vi "demo_Plug-in Open Source Library.vi"(11 "Stop Demo":refnum<user-event>) -> ()   [LabVIEW 2020]
panel:
  # "Open Source Library for FlexLogger Plug-ins\n\nA variety of community and NI contributed useful plug-ins written in LabVIEW for extending your FlexLogger Pro experience\n\nUse what's there or contribute your own!\n\nLook for 'Sequencer with Output Values' in FlexLogger Sessions\n\nhttps://github.com/ni/niflexlogger-plugins/tree/main/plugins"
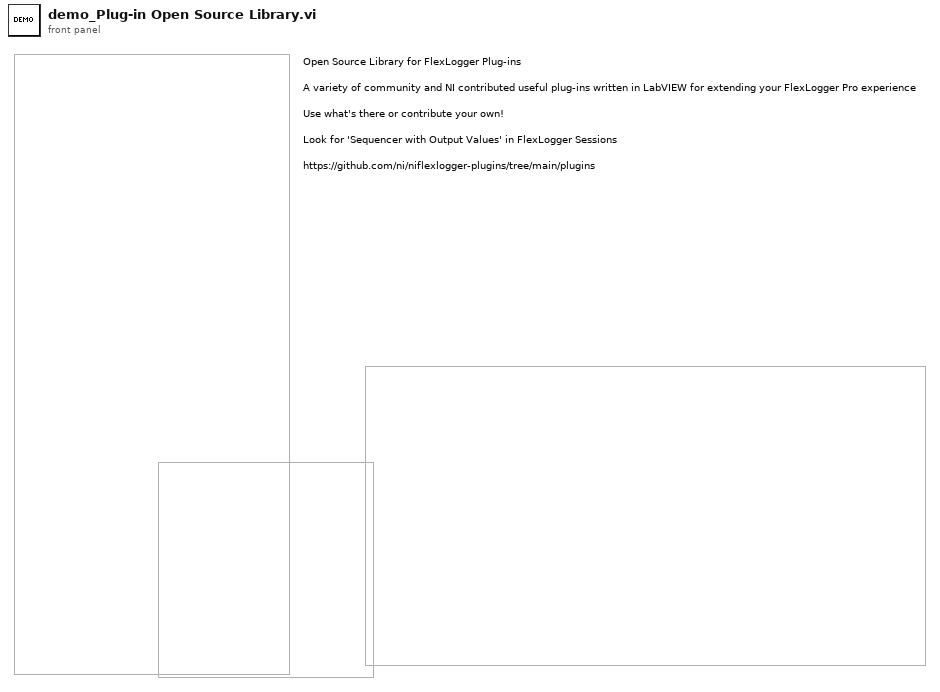
[diagram p1: front panel]
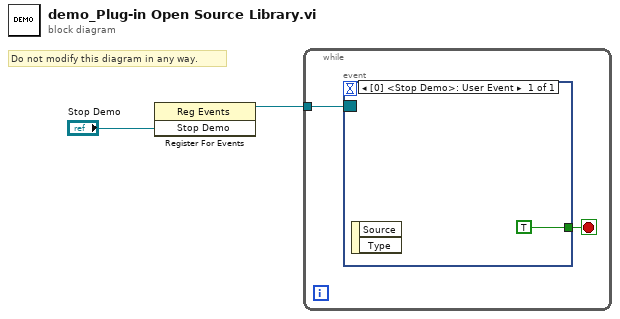
[diagram p0: block diagram]
diagram:
  # "Do not modify this diagram in any way."
  n1 = register-events("Stop Demo") -> (reference out=w1:refnum<event-registration>)  [unwired: 2 in, 1 out]
  n2 = while {
    tunnel: w1 -> [w4]
    stop <- w3 stop-if-true
    n3 = event shown="[0] <Stop Demo>: User Event" {
      selector: w4 -> [_]
      dyn-events: _ -> [_]
      timeout: _ -> [_]
      tunnel: [TRUE] -> w3
      event User Event {
        n4 = event-data() -> ()  [unwired: 1 in, 2 out]
      }
    }
  }
